vi "GetNumberOfItems.vi"(0 "reference in":refnum<class "Item.lvclass">, 5 "Error In":errorcluster) -> (14 "reference out":refnum<class "Item.lvclass">, 16 "ItemsInside":T1, 19 "Error Out":errorcluster)   [LabVIEW 2024, in "Item.lvclass"]
doc: "Get number of the item and convert it to map"
uses:
  Item.lvclass
  Items Inside Map.ctl
panel:
  # "Connector Pane"
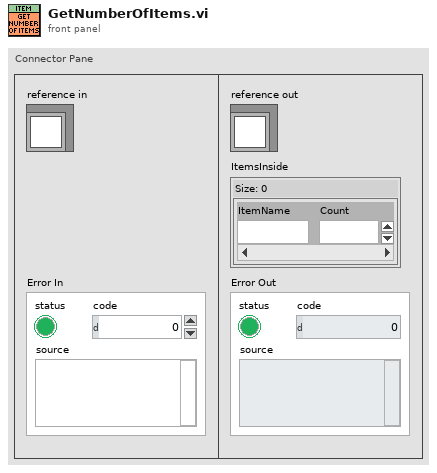
[diagram p1: front panel]
types:
  T1 = typedef "Items Inside Map.ctl" = map{string, u64}
  T2 = typedef "Item.lvclass/ObjectAttributes.ctl" = cluster{"Name":string, "Count":u64}
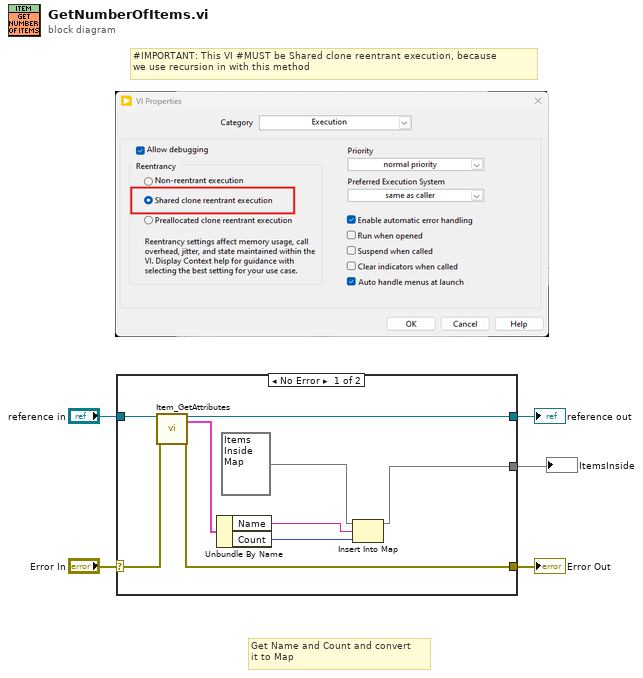
[diagram p0: block diagram]
diagram:
  # "#IMPORTANT: This VI #MUST be Shared clone reentrant execution, because\nwe use recursion in with this method"
  # "Get Name and Count and convert\nit to Map"
  n1 = case shown="No Error" "Error In" {
    selector: "Error In" -> [w14 w16]
    tunnel: [w12 w16] -> w4
    tunnel: [w10 w15] -> w2
    tunnel: "reference in" -> [w11 w15]
    tunnel: [w6 _] -> w1
    frame No Error {
      n2 = call "Item_GetAttributes.vi"("reference in"=w11, "Error In"=w14) -> ("reference out"=w10:refnum<class "Item.lvclass">, "Data"=w13:T2, "Error Out"=w12:errorcluster)  [unwired: 14 in, 1 out]
      n3 = Unbundle By Name(w13) -> ("Name"=w9:string, "Count"=w8:u64)
      n4 = Insert Into Map(map in=T1 {} ("ItemsInside"), key=w9, value=w8) -> (map out=w6:T1)  [unwired: 2 out]
    }
    frame Error {
    }
  }
  "Error Out" <- w4
  "reference out" <- w2
  "ItemsInside" <- w1
